vi "Write dt.vi"(8 "error in (no error)":errorcluster, 10 "dt CMD [s]":sgl, 11 "DCM-DSI-HW in":refnum<class "DCM-DSI.lvclass">) -> (0 "error out":errorcluster, 3 "DCM-DSI-HW out":refnum<class "DCM-DSI.lvclass">)   [LabVIEW 2016, in "DCM-DSI.lvclass"]
uses:
  DCM-DSI.lvclass
  DCM-DSI.lvclass/DCM-DSI.ctl
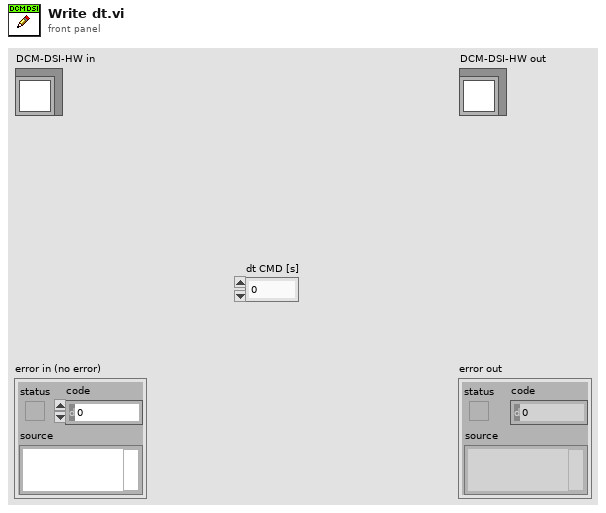
[diagram p1: front panel]
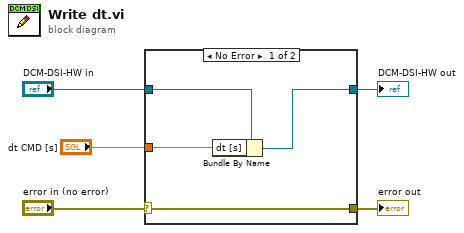
[diagram p0: block diagram]
diagram:
  n1 = case shown="No Error" "error in (no error)" {
    selector: "error in (no error)" -> [w9 w11]
    tunnel: [w9 w11] -> w4
    tunnel: [w7 w10] -> w2
    tunnel: "DCM-DSI-HW in" -> [w8 w10]
    tunnel: "dt CMD [s]" -> [w6 _]
    frame No Error {
      n2 = Bundle By Name(cluster=w8, "dt [s]"=w6) -> (w7:refnum<class "DCM-DSI.lvclass">)
    }
    frame Error {
    }
  }
  "error out" <- w4
  "DCM-DSI-HW out" <- w2
